vi "enum to string.vi"(10 "Deprecated":bool, 11 "enum in":variant) -> (2 "strings out":string[](array[string]), 3 "string out":string)   [LabVIEW 2019, in "Instrument.lvlib" / "Instrument.lvclass"]
doc: "Deprecated in favor of `Instrument-VIM.lvlib:enum to string.vim`"
uses:
  Instrument.lvclass
  c3e9e900-7d22-49c3-9fe5-275c32b7b2f3.vi
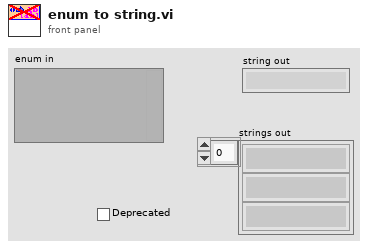
[diagram p1: front panel]
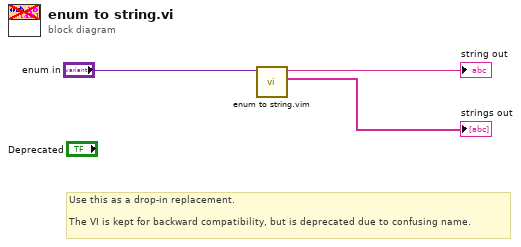
[diagram p0: block diagram]
diagram:
  # "Use this as a drop-in replacement.\n\nThe VI is kept for backward compatibility, but is deprecated due to confusing name."
  n1 = call "enum to string.vim"("enum in"="enum in") -> ("strings out"=→"strings out":string[], "string out"=→"string out":string)  [unwired: 9 in]
